vi "Initialize Camera.vi"(8 "error in (no error)":errorcluster, 11 "CCDCamera in":refnum<class "Simulated_CCD_Camera.lvclass">) -> (0 "error out":errorcluster, 3 "CCDCamera out":refnum<class "Simulated_CCD_Camera.lvclass">)   [LabVIEW 2018, in "Simulated_CCD_Camera.lvclass"]
uses:
  Simulated_CCD_Camera.lvclass
  Simulated_CCD_Camera.lvclass/Simulated_CCD_Camera.ctl
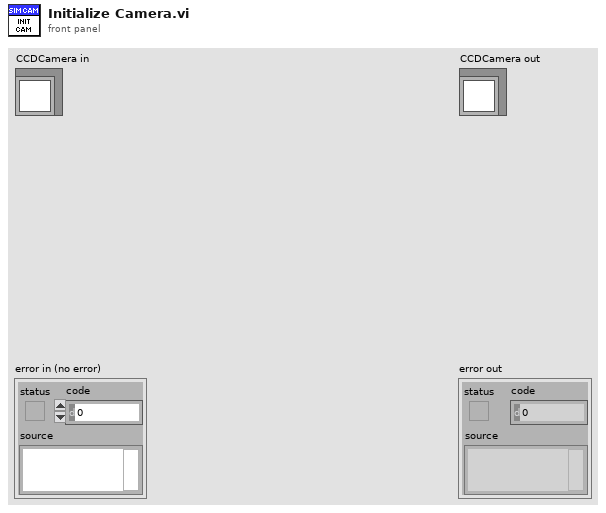
[diagram p1: front panel]
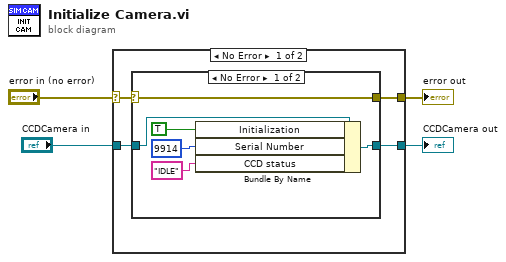
[diagram p0: block diagram]
diagram:
  n1 = case shown="No Error" "error in (no error)" {
    selector: "error in (no error)" -> [w8 w18]
    tunnel: [w6 w18] -> w1
    tunnel: [w7 w17] -> w2
    tunnel: "CCDCamera in" -> [w5 w17]
    frame No Error {
      n2 = case shown="No Error" w8 {
        selector: w8 -> [w13 w15]
        tunnel: w5 -> [w14 w16]
        tunnel: [w12 w16] -> w7
        tunnel: [w13 w15] -> w6
        frame No Error {
          n3 = Bundle By Name(cluster=w14, "Initialization"=TRUE, "Serial Number"=u16 9914 ("Initialization.Serial Number"), "CCD status"="IDLE" ("Camera Status.STATUS")) -> (w12:refnum<class "Simulated_CCD_Camera.lvclass">)
        }
        frame Error {
        }
      }
    }
    frame Error {
    }
  }
  "error out" <- w1
  "CCDCamera out" <- w2
